vi "LabVIEWInfos.vi"(8 "error in (no error)":errorcluster) -> (0 "error out":errorcluster, 3 "LabVIEW Info":T1[](array[typedef]))   [LabVIEW 2014]
uses:
  control/DEF-LabVIEW INFO.ctl
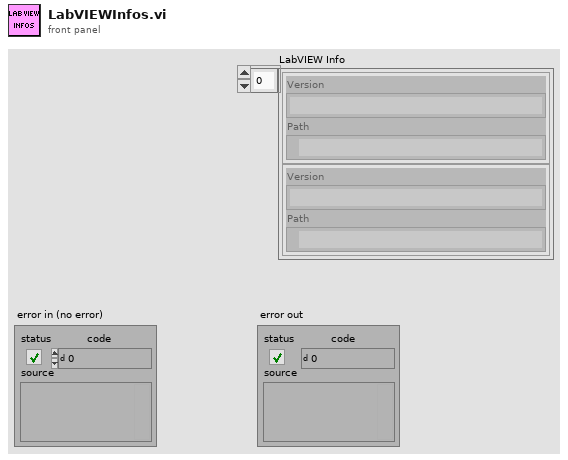
[diagram p1: front panel]
types:
  T1 = typedef "DEF-LabVIEW INFO.ctl" = cluster{"Version":string, "Path":path}
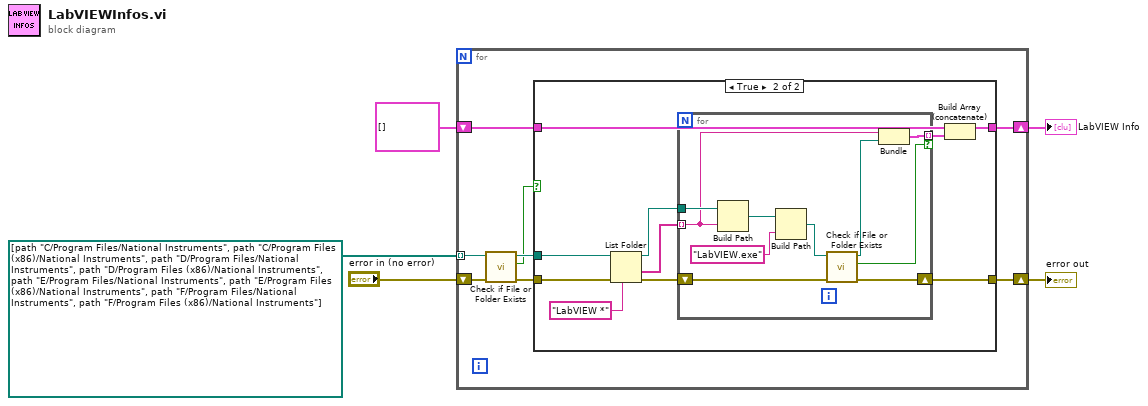
[diagram p0: block diagram]
diagram:
  n1 = for {
    tunnel: path[] [path "C:/Program Files/National Instruments", path "C:/Program Files (x86)/National Instruments", path "D:/Program Files/National Instruments", path "D:/Program Files (x86)/National Instruments", path "E:/Program Files/National Instruments", path "E:/Program Files (x86)/National Instruments", path "F:/Program Files/National Instruments", path "F:/Program Files (x86)/National Instruments"] -> [w13] mode=indexing
    shift-right: [w9] -> w3
    shift-left: T1[] [] ("LabVIEW Info") -> [w8]
    shift-right: [w7] -> w1
    shift-left: "error in (no error)" -> [w6]
    n2 = call <vilib>:"Check if File or Folder Exists.vi"("error in (no error)"=w6, "path"=w13) -> ("error out"=w11:errorcluster, "file or folder exists?"=w10:bool, "dup path"=w12:path)  [unwired: 7 in]
    n3 = case shown="True" w10 {
      tunnel: w12 -> [_ w18]
      tunnel: w11 -> [w14 w25]
      tunnel: [w15 w22] -> w9
      tunnel: w8 -> [w15 w21]
      tunnel: [w14 w20] -> w7
      frame False {
      }
      frame True {
        n4 = List Folder(path=w18, pattern="LabVIEW *", error in=w25) -> (path out=w17:path, folder names=w16:string[], error out=w24:errorcluster)  [unwired: 1 in, 1 out]
        n5 = for {
          tunnel: w17 -> [w35]
          tunnel: w16 -> [w30] mode=indexing
          tunnel: [w28] -> w23 mode=indexing if=w29
          shift-right: [w26] -> w20
          shift-left: w24 -> [w34]
          n6 = Build Path(base path=w35, name or relative path=w30) -> (appended path=w33:path)
          n7 = Build Path(base path=w33, name or relative path="LabVIEW.exe") -> (appended path=w31:path)
          n8 = call <vilib>:"Check if File or Folder Exists.vi"("error in (no error)"=w34, "path"=w31) -> ("error out"=w26:errorcluster, "file or folder exists?"=w29:bool, "dup path"=w27:path)  [unwired: 7 in]
          n9 = Bundle(w30, "dup path"=w27) -> (w28:cluster{string, "dup path":path})  [unwired: 1 in]
        }
        n10 = Build Array (concatenate)(w21, w23) -> (w22:T1[])
      }
    }
  }
  "LabVIEW Info" <- w3
  "error out" <- w1
